vi "edittest read fields from file.vi"(8 "error in (no error)":errorcluster, 9 "Version":string, 11 "File Refnum In":T4) -> (0 "error out":errorcluster, 2 "Sequence Fields":T1[](array[typedef]), 3 "File Refnum Out":T4)   [LabVIEW 2011]
uses:
  <vilib>/Utility/config.llb/Config Data RefNum.ctl
  server/database/Fields/Field Record.ctl
  server/database/Fields/Field DataTypes.ctl
  server/database/Fields/Field NextItem.ctl
  <vilib>/Utility/config.llb/Read Key (I32).vi
  <vilib>/Utility/config.llb/Read Key (String).vi
  <vilib>/Utility/config.llb/NI_LVConfig.lvlib
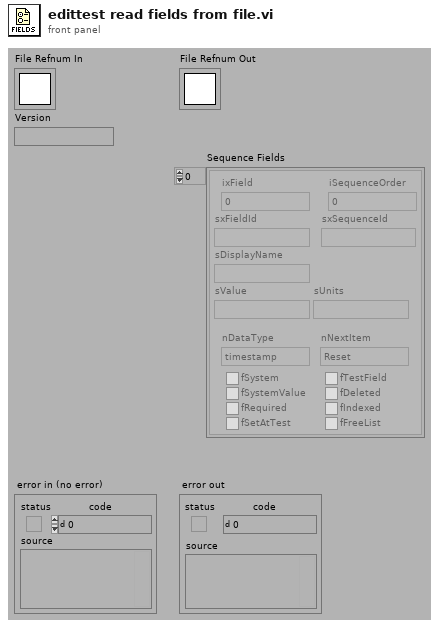
[diagram p1: front panel]
types:
  T1 = typedef "Field Record.ctl" = cluster{"ixField":i32, "iSequenceOrder":i32, "sxFieldId":string, "sxSequenceId":string, "sDisplayName":string, "sValue":string, "sUnits":string, "nDataType":T2, "nNextItem":T3, "fSystem":bool, "fSystemValue":bool, "fRequired":bool, "fSetAtTest":bool, "fTestField":bool, "fDeleted":bool, "fIndexed":bool, "fFreeList":bool}
  T2 = typedef "Field DataTypes.ctl" = enum32{"text", "numeric", "list", "timestamp", "boolean"}
  T3 = typedef "Field NextItem.ctl" = enum32{"Reset", "Retain", "Auto-Increment"}
  T4 = typedef "NI_LVConfig.lvlib/Config Data RefNum.ctl" = refnum<k1>
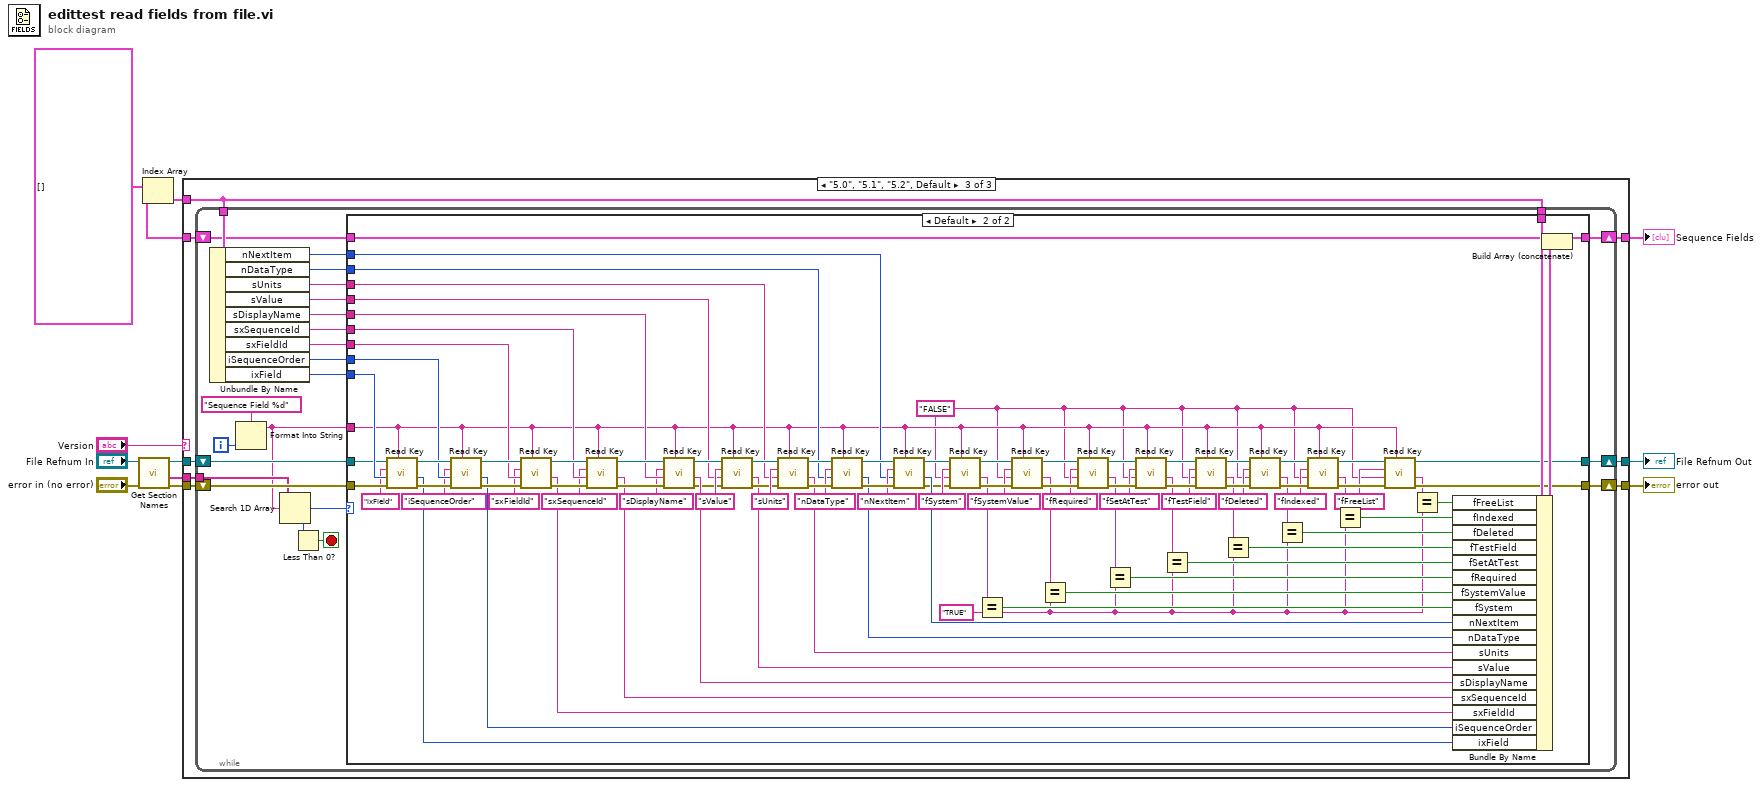
[diagram p0: block diagram]
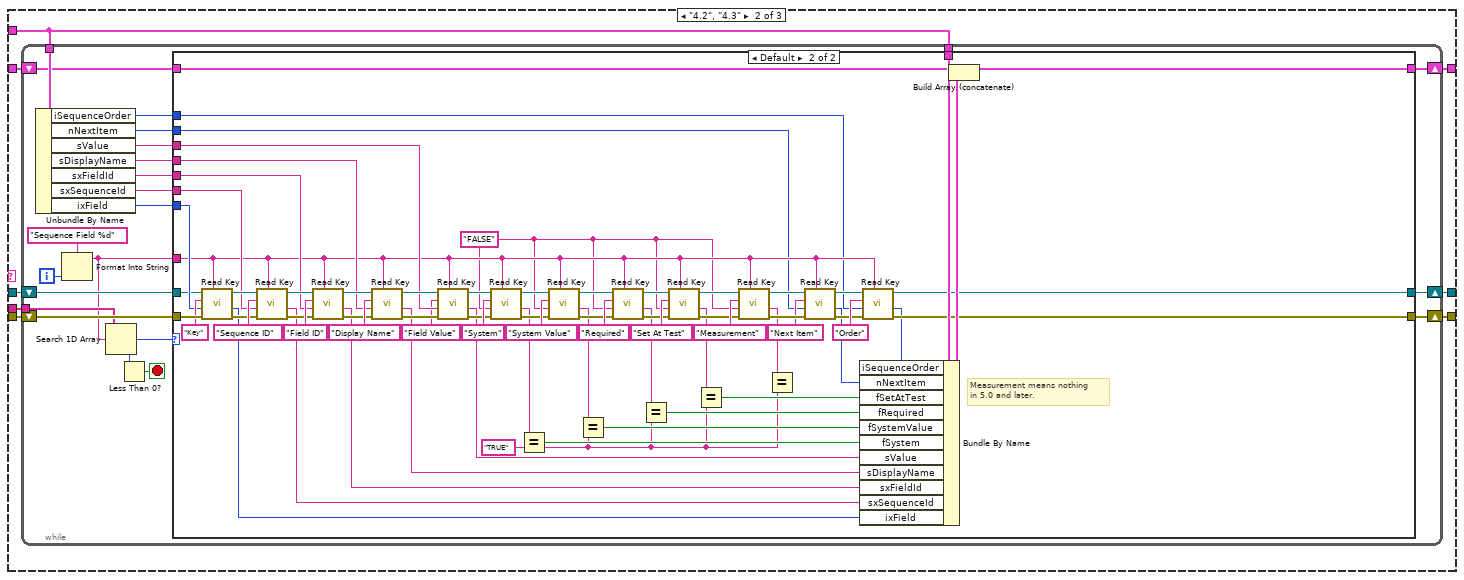
[diagram p3: hidden frame]
diagram:
  w3 = T1[] [] ("Sequence Fields")
  n1 = call <vilib>:"Get Section Names.vi"("error in (no error)"="error in (no error)", "refnum"="File Refnum In") -> ("error out"=w11:errorcluster, "section names"=w9:string[], "refnum out"=w10:T4)  [unwired: 7 out]
  n2 = Index Array(array=w3) -> (element=w8:T1)  [unwired: 1 in]
  n3 = case shown="\"5.0\", \"5.1\", \"5.2\", Default" "Version" {
    tunnel: w11 -> [w12 w21 w121]
    tunnel: w10 -> [w13 w20 w120]
    tunnel: w9 -> [_ w19 w119]
    tunnel: w8 -> [_ w14 w118]
    tunnel: [w13 w18 w117] -> w5
    tunnel: [w12 w17 w116] -> w4
    tunnel: w3 -> [_ w16 w115]
    tunnel: [_ w15 w114] -> w2
    frame "-1.0" {
    }
    frame "4.2", "4.3" {
      n4 = while {
        shift-right: [w38] -> w18
        shift-left: w20 -> [w30]
        shift-right: [w39] -> w17
        shift-left: w21 -> [w40]
        tunnel: w14 -> [w37]
        tunnel: w14 -> [w31]
        tunnel: w19 -> [w29]
        shift-right: [w24] -> w15
        shift-left: w16 -> [w25]
        i -> [w41]
        stop <- w26 stop-if-true
        n5 = Unbundle By Name(w37) -> ("iSequenceOrder"=w23:i32, "nNextItem"=w22:T3, "sValue"=w32:string, "sDisplayName"=w33:string, "sxFieldId"=w34:string, "sxSequenceId"=w35:string, "ixField"=w36:i32)
        n6 = Format Into String(format string="Sequence Field %d", w41) -> (resulting string=w28:string)  [unwired: 2 in, 1 out]
        n7 = Search 1D Array(1D array=w29, element=w28) -> (index of element=w27:i32)  [unwired: 1 out]
        n8 = Less Than 0?(x=w27) -> (x < 0?=w26:bool)
        n9 = case shown="Default" w27 {
          tunnel: w40 -> [w45 w113]
          tunnel: w28 -> [_ w63]
          tunnel: [w45 w68] -> w39
          tunnel: [w44 w67] -> w38
          tunnel: w36 -> [_ w91]
          tunnel: w35 -> [_ w90]
          tunnel: w34 -> [_ w89]
          tunnel: w33 -> [_ w88]
          tunnel: w32 -> [_ w87]
          tunnel: w31 -> [_ w86]
          tunnel: w30 -> [w44 w80]
          tunnel: w25 -> [w43 w79]
          tunnel: [w43 w77] -> w24
          tunnel: w23 -> [_ w62]
          tunnel: w22 -> [_ w47]
          frame -1 {
          }
          frame Default {
            w48 = "FALSE"
            w46 = "TRUE"
            # "Measurement means nothing\nin 5.0 and later."
            n10 = call-poly <vilib>:"Read Key.vi"("section"=w63, "error in (no error)"=w113, "default value"=w91, "key"="Key", "refnum"=w80) -> ("error out"=w106:errorcluster, "value"=w85:i32, "refnum out"=w97:T4)  [unwired: 4 out]
            n11 = call-poly <vilib>:"Read Key.vi"("section"=w63, "error in (no error)"=w106, "default value"=w90, "key"="Sequence ID", "refnum"=w97) -> ("error out"=w105:errorcluster, "value"=w84:string, "refnum out"=w98:T4)  [unwired: 1 in, 3 out]
            n12 = call-poly <vilib>:"Read Key.vi"("section"=w63, "error in (no error)"=w105, "default value"=w89, "key"="Field ID", "refnum"=w98) -> ("error out"=w92:errorcluster, "value"=w83:string, "refnum out"=w93:T4)  [unwired: 1 in, 3 out]
            n13 = call-poly <vilib>:"Read Key.vi"("section"=w63, "error in (no error)"=w92, "default value"=w88, "key"="Display Name", "refnum"=w93) -> ("error out"=w95:errorcluster, "value"=w82:string, "refnum out"=w94:T4)  [unwired: 1 in, 3 out]
            n14 = call-poly <vilib>:"Read Key.vi"("section"=w63, "error in (no error)"=w95, "default value"=w87, "key"="Field Value", "refnum"=w94) -> ("error out"=w104:errorcluster, "value"=w81:string, "refnum out"=w99:T4)  [unwired: 1 in, 3 out]
            n15 = call-poly <vilib>:"Read Key.vi"("section"=w63, "error in (no error)"=w104, "default value"=w48, "key"="System", "refnum"=w99) -> ("error out"=w103:errorcluster, "value"=w54:string, "refnum out"=w100:T4)  [unwired: 1 in, 3 out]
            n16 = Equal?(x=w54, y=w46) -> (x = y?=w53:bool)
            n17 = call-poly <vilib>:"Read Key.vi"("section"=w63, "error in (no error)"=w103, "default value"=w48, "key"="System Value", "refnum"=w100) -> ("error out"=w102:errorcluster, "value"=w55:string, "refnum out"=w101:T4)  [unwired: 1 in, 3 out]
            n18 = Equal?(x=w55, y=w46) -> (x = y?=w52:bool)
            n19 = call-poly <vilib>:"Read Key.vi"("section"=w63, "error in (no error)"=w102, "default value"=w48, "key"="Required", "refnum"=w101) -> ("error out"=w72:errorcluster, "value"=w50:string, "refnum out"=w73:T4)  [unwired: 1 in, 3 out]
            n20 = Equal?(x=w50, y=w46) -> (x = y?=w49:bool)
            n21 = call-poly <vilib>:"Read Key.vi"("section"=w63, "error in (no error)"=w72, "default value"=w48, "key"="Set At Test", "refnum"=w73) -> ("error out"=w71:errorcluster, "value"=w56:string, "refnum out"=w64:T4)  [unwired: 1 in, 3 out]
            n22 = Equal?(x=w56, y=w46) -> (x = y?=w51:bool)
            n23 = call-poly <vilib>:"Read Key.vi"("section"=w63, "error in (no error)"=w71, "default value"=w48, "key"="Measurement", "refnum"=w64) -> ("error out"=w70:errorcluster, "value"=w57:string, "refnum out"=w65:T4)  [unwired: 1 in, 3 out]
            n24 = Equal?(x=w57, y=w46) -> ()  [unwired: 1 out]
            n25 = call-poly <vilib>:"Read Key.vi"("section"=w63, "error in (no error)"=w70, "default value"=w47, "key"="Next Item", "refnum"=w65) -> ("error out"=w69:errorcluster, "value"=w58:i32, "refnum out"=w66:T4)  [unwired: 4 out]
            n26 = call-poly <vilib>:"Read Key.vi"("section"=w63, "error in (no error)"=w69, "default value"=w62, "key"="Order", "refnum"=w66) -> ("error out"=w68:errorcluster, "value"=w60:i32, "refnum out"=w67:T4)  [unwired: 4 out]
            n27 = Bundle By Name(cluster=w86, "iSequenceOrder"=w60, "nNextItem"=w58, "fSetAtTest"=w51, "fRequired"=w49, "fSystemValue"=w52, "fSystem"=w53, "sValue"=w81, "sDisplayName"=w82, "sxFieldId"=w83, "sxSequenceId"=w84, "ixField"=w85) -> (w78:T1)
            n28 = Build Array (concatenate)(w79, w78) -> (w77:T1[])
          }
        }
      }
    }
    frame "5.0", "5.1", "5.2", Default {
      n29 = while {
        shift-right: [w140] -> w117
        shift-left: w120 -> [w132]
        shift-right: [w141] -> w116
        shift-left: w121 -> [w142]
        tunnel: w118 -> [w139]
        tunnel: w118 -> [w133]
        tunnel: w119 -> [w131]
        shift-right: [w126] -> w114
        shift-left: w115 -> [w127]
        i -> [w143]
        stop <- w128 stop-if-true
        n30 = Unbundle By Name(w139) -> ("nNextItem"=w123:T3, "nDataType"=w122:T2, "sUnits"=w125:string, "sValue"=w124:string, "sDisplayName"=w134:string, "sxSequenceId"=w135:string, "sxFieldId"=w136:string, "iSequenceOrder"=w137:i32, "ixField"=w138:i32)
        n31 = Format Into String(format string="Sequence Field %d", w143) -> (resulting string=w130:string)  [unwired: 2 in, 1 out]
        n32 = Search 1D Array(1D array=w131, element=w130) -> (index of element=w129:i32)  [unwired: 1 out]
        n33 = Less Than 0?(x=w129) -> (x < 0?=w128:bool)
        n34 = case shown="Default" w129 {
          tunnel: w142 -> [w147 w241]
          tunnel: w130 -> [_ w164]
          tunnel: [w147 w162] -> w141
          tunnel: [w146 w163] -> w140
          tunnel: w138 -> [_ w228]
          tunnel: w137 -> [_ w227]
          tunnel: w136 -> [_ w226]
          tunnel: w135 -> [_ w225]
          tunnel: w134 -> [_ w224]
          tunnel: w133 -> [_ w223]
          tunnel: w132 -> [w146 w217]
          tunnel: w127 -> [w145 w216]
          tunnel: [w145 w214] -> w126
          tunnel: w125 -> [_ w182]
          tunnel: w124 -> [_ w183]
          tunnel: w123 -> [_ w176]
          tunnel: w122 -> [_ w177]
          frame -1 {
          }
          frame Default {
            w159 = "FALSE"
            w148 = "TRUE"
            n35 = call-poly <vilib>:"Read Key.vi"("section"=w164, "error in (no error)"=w241, "default value"=w228, "key"="ixField", "refnum"=w217) -> ("error out"=w240:errorcluster, "value"=w222:i32, "refnum out"=w233:T4)  [unwired: 4 out]
            n36 = call-poly <vilib>:"Read Key.vi"("section"=w164, "error in (no error)"=w240, "default value"=w227, "key"="iSequenceOrder", "refnum"=w233) -> ("error out"=w239:errorcluster, "value"=w221:i32, "refnum out"=w234:T4)  [unwired: 4 out]
            n37 = call-poly <vilib>:"Read Key.vi"("section"=w164, "error in (no error)"=w239, "default value"=w226, "key"="sxFieldId", "refnum"=w234) -> ("error out"=w229:errorcluster, "value"=w220:string, "refnum out"=w230:T4)  [unwired: 1 in, 3 out]
            n38 = call-poly <vilib>:"Read Key.vi"("section"=w164, "error in (no error)"=w229, "default value"=w225, "key"="sxSequenceId", "refnum"=w230) -> ("error out"=w232:errorcluster, "value"=w219:string, "refnum out"=w231:T4)  [unwired: 1 in, 3 out]
            n39 = call-poly <vilib>:"Read Key.vi"("section"=w164, "error in (no error)"=w232, "default value"=w224, "key"="sDisplayName", "refnum"=w231) -> ("error out"=w193:errorcluster, "value"=w218:string, "refnum out"=w194:T4)  [unwired: 1 in, 3 out]
            n40 = call-poly <vilib>:"Read Key.vi"("section"=w164, "error in (no error)"=w193, "default value"=w183, "key"="sValue", "refnum"=w194) -> ("error out"=w188:errorcluster, "value"=w181:string, "refnum out"=w189:T4)  [unwired: 1 in, 3 out]
            n41 = call-poly <vilib>:"Read Key.vi"("section"=w164, "error in (no error)"=w188, "default value"=w182, "key"="sUnits", "refnum"=w189) -> ("error out"=w187:errorcluster, "value"=w180:string, "refnum out"=w190:T4)  [unwired: 1 in, 3 out]
            n42 = call-poly <vilib>:"Read Key.vi"("section"=w164, "error in (no error)"=w187, "default value"=w177, "key"="nDataType", "refnum"=w190) -> ("error out"=w186:errorcluster, "value"=w179:i32, "refnum out"=w191:T4)  [unwired: 4 out]
            n43 = call-poly <vilib>:"Read Key.vi"("section"=w164, "error in (no error)"=w186, "default value"=w176, "key"="nNextItem", "refnum"=w191) -> ("error out"=w173:errorcluster, "value"=w178:i32, "refnum out"=w174:T4)  [unwired: 4 out]
            n44 = call-poly <vilib>:"Read Key.vi"("section"=w164, "error in (no error)"=w173, "default value"=w159, "key"="fSystem", "refnum"=w174) -> ("error out"=w238:errorcluster, "value"=w202:string, "refnum out"=w235:T4)  [unwired: 1 in, 3 out]
            n45 = Equal?(x=w202, y=w148) -> (x = y?=w149:bool)
            n46 = call-poly <vilib>:"Read Key.vi"("section"=w164, "error in (no error)"=w238, "default value"=w159, "key"="fSystemValue", "refnum"=w235) -> ("error out"=w237:errorcluster, "value"=w203:string, "refnum out"=w236:T4)  [unwired: 1 in, 3 out]
            n47 = Equal?(x=w203, y=w148) -> (x = y?=w150:bool)
            n48 = call-poly <vilib>:"Read Key.vi"("section"=w164, "error in (no error)"=w237, "default value"=w159, "key"="fRequired", "refnum"=w236) -> ("error out"=w212:errorcluster, "value"=w201:string, "refnum out"=w213:T4)  [unwired: 1 in, 3 out]
            n49 = Equal?(x=w201, y=w148) -> (x = y?=w151:bool)
            n50 = call-poly <vilib>:"Read Key.vi"("section"=w164, "error in (no error)"=w212, "default value"=w159, "key"="fSetAtTest", "refnum"=w213) -> ("error out"=w211:errorcluster, "value"=w204:string, "refnum out"=w206:T4)  [unwired: 1 in, 3 out]
            n51 = Equal?(x=w204, y=w148) -> (x = y?=w152:bool)
            n52 = call-poly <vilib>:"Read Key.vi"("section"=w164, "error in (no error)"=w211, "default value"=w159, "key"="fTestField", "refnum"=w206) -> ("error out"=w210:errorcluster, "value"=w205:string, "refnum out"=w207:T4)  [unwired: 1 in, 3 out]
            n53 = Equal?(x=w205, y=w148) -> (x = y?=w153:bool)
            n54 = call-poly <vilib>:"Read Key.vi"("section"=w164, "error in (no error)"=w210, "default value"=w159, "key"="fDeleted", "refnum"=w207) -> ("error out"=w209:errorcluster, "value"=w166:string, "refnum out"=w208:T4)  [unwired: 1 in, 3 out]
            n55 = Equal?(x=w166, y=w148) -> (x = y?=w154:bool)
            n56 = call-poly <vilib>:"Read Key.vi"("section"=w164, "error in (no error)"=w209, "default value"=w159, "key"="fIndexed", "refnum"=w208) -> ("error out"=w161:errorcluster, "value"=w157:string, "refnum out"=w165:T4)  [unwired: 1 in, 3 out]
            n57 = Equal?(x=w157, y=w148) -> (x = y?=w155:bool)
            n58 = call-poly <vilib>:"Read Key.vi"("section"=w164, "error in (no error)"=w161, "default value"=w159, "key"="fFreeList", "refnum"=w165) -> ("error out"=w162:errorcluster, "value"=w158:string, "refnum out"=w163:T4)  [unwired: 1 in, 3 out]
            n59 = Equal?(x=w158, y=w148) -> (x = y?=w156:bool)
            n60 = Bundle By Name(cluster=w223, "fFreeList"=w156, "fIndexed"=w155, "fDeleted"=w154, "fTestField"=w153, "fSetAtTest"=w152, "fRequired"=w151, "fSystemValue"=w150, "fSystem"=w149, "nNextItem"=w178, "nDataType"=w179, "sUnits"=w180, "sValue"=w181, "sDisplayName"=w218, "sxSequenceId"=w219, "sxFieldId"=w220, "iSequenceOrder"=w221, "ixField"=w222) -> (w215:T1)
            n61 = Build Array (concatenate)(w216, w215) -> (w214:T1[])
          }
        }
      }
    }
  }
  "error out" <- w4
  "File Refnum Out" <- w5
  "Sequence Fields" <- w2
